vi "Extract Decoration Text.vi"(8 "error in (no error)":errorcluster, 10 "VI Ref in":refnum<vi>, 11 "VI Data in":refnum<class "VI Data.lvclass">) -> (0 "error out":errorcluster, 2 "VI Ref out":refnum<vi>, 3 "VI Data out":refnum<class "VI Data.lvclass">)   [LabVIEW 2013, in "SET Project Data.lvlib" / "VI Data.lvclass"]
uses:
  VI Data.lvclass
  <vilib>/Utility/traverseref.llb/TRef TravTarget.ctl
  VI Data.lvclass/VI Data.ctl
  Control Classes/GObject/GObject.lvclass
  <vilib>/Utility/traverseref.llb/VI Scripting - Traverse.lvlib
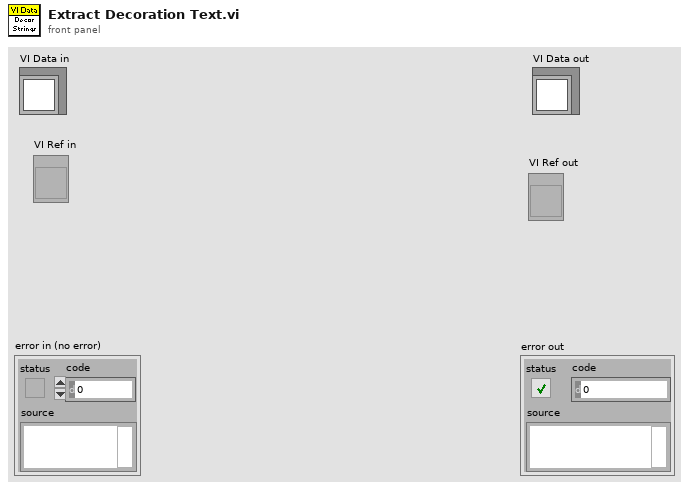
[diagram p1: front panel]
types:
  T1 = typedef "TRef TravTarget.ctl" = enum16{"FP", "BD", "Other"}
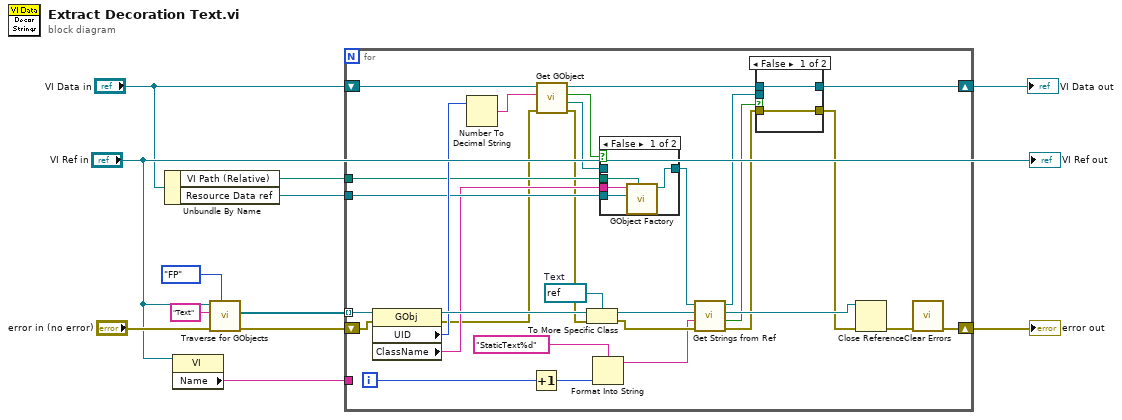
[diagram p0: block diagram]
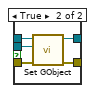
[diagram p2: hidden frame]
diagram:
  n1 = Unbundle By Name("VI Data in") -> ("VI Path (Relative)"=w3:path, "Resource Data ref"=w4:refnum<data-value>)
  n2 = property class="VI"(reference="VI Ref in") -> ("Name"=w5:string)  [unwired: 1 in, 2 out]
  n3 = call <vilib>:"Traverse for GObjects.vi"("Traverse Target"=TRef_TravTarget."FP", "error in (no error)"="error in (no error)", "Class Name"="Text", "VI Refnum"="VI Ref in") -> ("error out"=w9:errorcluster, "References"=w10:refnum<vi>[])  [unwired: 4 in, 2 out]
  n4 = for {
    tunnel: w10 -> [w31] mode=indexing
    shift-right: [w36] -> w7
    shift-left: w9 -> [w30]
    tunnel: w4 -> [w24]
    tunnel: w5 -> [_]
    tunnel: w3 -> [w22]
    shift-right: [w19] -> w1
    shift-left: "VI Data in" -> [w32]
    i -> [w38]
    w42 = refnum<vi> refnum  # Text
    n5 = property class="GObj"(reference=w31, error in=w30) -> (reference out=w29:refnum<vi>, error out=w16:errorcluster, "UID"=w28:i32, "ClassName"=w23:string)
    n6 = Number To Decimal String(number=w28) -> (decimal integer string=w27:string)  [unwired: 1 in]
    n7 = Increment(x=w38) -> (x+1=w35:i32)
    n8 = call-dynamic "Get GObject.vi"("error in (no error)"=w16, "GObject UID"=w27, "VI Data in"=w32) -> ("error out"=w15:errorcluster, "GObject"=w25:refnum<class "GObject.lvclass">, "found"=w26:bool, "VI Data out"=w20:refnum<class "VI Data.lvclass">)  [unwired: 5 in]
    n9 = To More Specific Class(target class=w42, reference=w29, error in=w15) -> (specific class reference=w41:refnum<vi>, error out=w40:errorcluster)
    n10 = Format Into String(format string="StaticText%d", w35) -> (resulting string=w34:string)  [unwired: 2 in, 1 out]
    n11 = case shown="False" w26 {
      tunnel: w25 -> [_ w54]
      tunnel: [w53 w54] -> w21
      tunnel: w24 -> [w52 _]
      tunnel: w23 -> [w51 _]
      tunnel: w22 -> [w50 _]
      frame False {
        n12 = call "GObject Factory.vi"("Owning VI"=w50, "LangFile ref"=w52, "ClassName"=w51) -> ("GObject"=w53:refnum<class "GObject.lvclass">)  [unwired: 8 in]
      }
      frame True {
      }
    }
    n13 = call-dynamic "Get Strings from Ref.vi"("error in (no error)"=w40, "Label Prefix"=w34, "GObj Refnum in"=w41, "GObject in"=w21) -> ("error out"=w14:errorcluster, "Valid?"=w18:bool, "GObj Refnum out"=w37:refnum<vi>, "GObject out"=w17:refnum<class "GObject.lvclass">)  [unwired: 3 in, 1 out]
    n14 = case shown="False" w18 {
      tunnel: w20 -> [w44 w49]
      tunnel: [w44 w48] -> w19
      tunnel: w17 -> [_ w47]
      tunnel: [w43 w46] -> w13
      tunnel: w14 -> [w43 w45]
      frame False {
      }
      frame True {
        n15 = call "Set GObject.vi"("error in (no error)"=w45, "GObject.lvclass"=w47, "VI Data in"=w49) -> ("error out"=w46:errorcluster, "VI Data out"=w48:refnum<class "VI Data.lvclass">)  [unwired: 6 in, 1 out]
      }
    }
    n16 = Close Reference(reference=w37, error in (no error)=w13) -> (error out=w33:errorcluster)
    n17 = call <vilib>:"Clear Errors.vi"("error in (no error)"=w33) -> ("error out"=w36:errorcluster)  [unwired: 6 in]
  }
  "error out" <- w7
  "VI Data out" <- w1
  "VI Ref out" <- "VI Ref in"
